vi "Directory to Tree.vi"(4 "Files found":i32(listbox)=1, 6 "error in":errorcluster, 7 "Pattern":string, 8 "Path to start the search":path, 9 "Tree In":refnum<vi>) -> (0 "error out":errorcluster, 1 "Array of files found":path[](array[path]), 2 "Number of files found":i32, 3 "Tree Out":refnum<vi>)   [LabVIEW 2012]
doc: "This VI searches \"Path to start the search\" and all the path's subdirectories for files having names specified in \"Pattern to search\". This VI specifically does not search Windows shortcuts."
panel:
  in  "Parent Tag":string
  out "Working":bool=TRUE
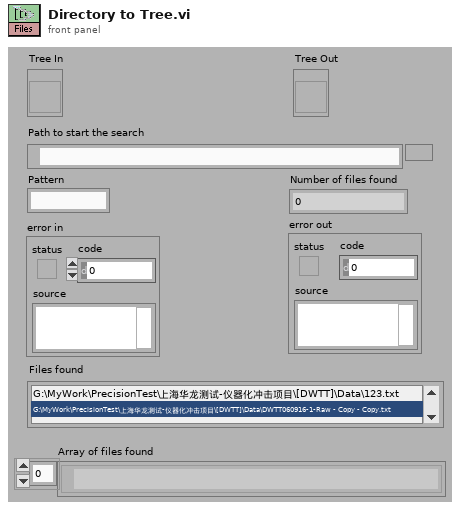
[diagram p1: front panel]
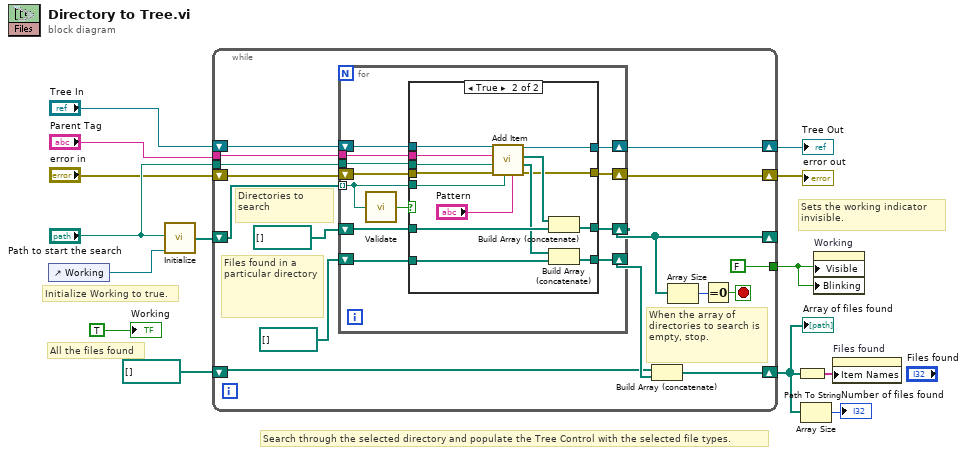
[diagram p0: block diagram]
diagram:
  # "Search through the selected directory and populate the Tree Control with the selected file types."
  # "Initialize Working to true."
  # "All the files found"
  # "Sets the working indicator invisible."
  n1 = control-ref of="Working"() -> (w6:refnum<vi>)
  n2 = call "Initialize.vi"("Working"=w6, "Path to start the search"="Path to start the search") -> ("Array"=w14:path[])  [unwired: 2 in]
  n3 = while {
    shift-right: [w28] -> _
    shift-left: w14 -> [w24]
    shift-right: [w29] -> w11
    shift-left: path[] [] -> [w22]
    tunnel: [FALSE] -> w8
    tunnel: "Parent Tag" -> [w19]
    tunnel: "Path to start the search" -> [w18]
    shift-right: [w15] -> w1
    shift-left: "error in" -> [w17]
    shift-right: [w16] -> w2
    shift-left: "Tree In" -> [w20]
    stop <- w27 stop-if-true
    # "When the array of directories to search is empty, stop."
    # "Files found in a particular directory"
    # "Directories to search"
    n4 = for {
      tunnel: w24 -> [w38] mode=indexing
      shift-right: [w42] -> w28
      shift-left: path[] [] -> [w41]
      shift-right: [w39] -> w23
      shift-left: path[] [] -> [w40]
      tunnel: w19 -> [w35]
      tunnel: w18 -> [w34]
      shift-right: [w31] -> w15
      shift-left: w17 -> [w33]
      shift-right: [w32] -> w16
      shift-left: w20 -> [w36]
      n5 = call "Validate.vi"("Path"=w38) -> ("Valid Path?"=w37:bool)
      n6 = case shown="True" w37 {
        tunnel: [w46 w60] -> w42
        tunnel: w41 -> [w46 w59]
        tunnel: w40 -> [w45 w58]
        tunnel: [w45 w57] -> w39
        tunnel: w38 -> [_ w55]
        tunnel: w36 -> [w44 w50]
        tunnel: w35 -> [_ w48]
        tunnel: w34 -> [_ w47]
        tunnel: [w44 w49] -> w32
        tunnel: [w43 w51] -> w31
        tunnel: w33 -> [w43 w52]
        frame False {
          # "This file is either a shortcut or not a path"
        }
        frame True {
          n7 = call "Add Item.vi"("Pattern"="Pattern", "Path"=w55, "error in"=w52, "Path to start the search"=w47, "Parent Tag"=w48, "Tree In"=w50) -> ("error out"=w51:errorcluster, "Files Found"=w53:path[], "Folders Found"=w54:path[], "Tree Out"=w49:refnum<vi>)  [unwired: 1 in]
          n8 = Build Array (concatenate)(w54, w59) -> (w60:path[])
          n9 = Build Array (concatenate)(w53, w58) -> (w57:path[])
        }
      }
    }
    n10 = Build Array (concatenate)(w22, w23) -> (w29:path[])
    n11 = Array Size(array=w28) -> (size(s)=w30:i32)
    n12 = Equal To 0?(x=w30) -> (x = 0?=w27:bool)
  }
  "Array of files found" <- w11
  "error out" <- w1
  "Tree Out" <- w2
  n13 = Path To String(path=w11) -> (string=w13:string[])
  n14 = Array Size(array=w11) -> (size(s)=→"Number of files found":i32)
  n15 = property on="Working" class="Bool (strict)"("Visible"=w8, "Blinking"=w8) -> ()  [unwired: 2 in, 2 out]
  n16 = property on="Files found" class="LstBox (strict)"("Item Names"=w13) -> ()  [unwired: 2 in, 2 out]
  "Working" <- TRUE
